vi "Variable list PSU analog.vi"() -> (6 "Variant":variant, 10 "Array":T1[](array[typedef]) {"Default Scaling"."Offset" format="%.5f"; "Default Scaling"."Gain" format="%.5f"})   [LabVIEW 2011]
uses:
  Measurments Handling/Fixed Analog Channel Definition.ctl
  Measurments Handling/Units/Quantity enum.ctl
  Measurments Handling/Update frequensies.ctl
  Measurments Handling/Channel catagory Enum.ctl
  Measurments Handling/Scaling.ctl
  Measurments Handling/Channel Classification Enum.ctl
  Measurments Handling/Common/Variable List Common Analog.ctl
  <vilib>/Utility/VariantDataType/GetNumericInfo.vi
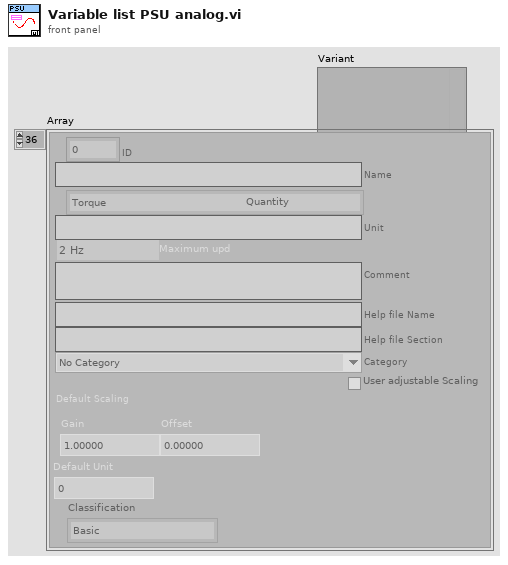
[diagram p1: front panel]
types:
  T1 = typedef "Fixed Analog Channel Definition.ctl" = cluster{"ID":u16, "Name":string, "Quantity":T2, "Unit":string, "Maximum upd":T3, "Comment":string, "Help file Name":string, "Help file Section ":string, "Category":T4, "User adjustable Scaling":bool, "Default Scaling":T5, "Default Unit":i32, "Classification":T6}
  T2 = typedef "Quantity enum.ctl" = enum16{"NA", "Acceleration", "Angle", "Current", "Force", "Distance", "Pressure", "Resistance", "Rotational Speed", "Speed", "Temperature", "Tension", "Torque", "Voltage", "Weight"}
  T3 = typedef "Update frequensies.ctl" = enum16{"2 Hz", "1 Hz", "0.1 Hz"}
  T4 = typedef "Channel catagory Enum.ctl" = enum16{"No Category", "Power", "Temperature", "Pressure"}
  T5 = typedef "Scaling.ctl" = cluster{"Gain":dbl, "Offset":dbl}
  T6 = typedef "Channel Classification Enum.ctl" = enum16{"Basic", "Advanced", "Expert", "Unused"}
  T7 = typedef "Variable List Common Analog.ctl" = enum16{"HVPSU Head Voltage", "HVPSU TS Voltage", "HVPSU Current", "PCP Cable Resistance", "Winch Depth", "Winch Line Speed", "Winch Wire Tension"}
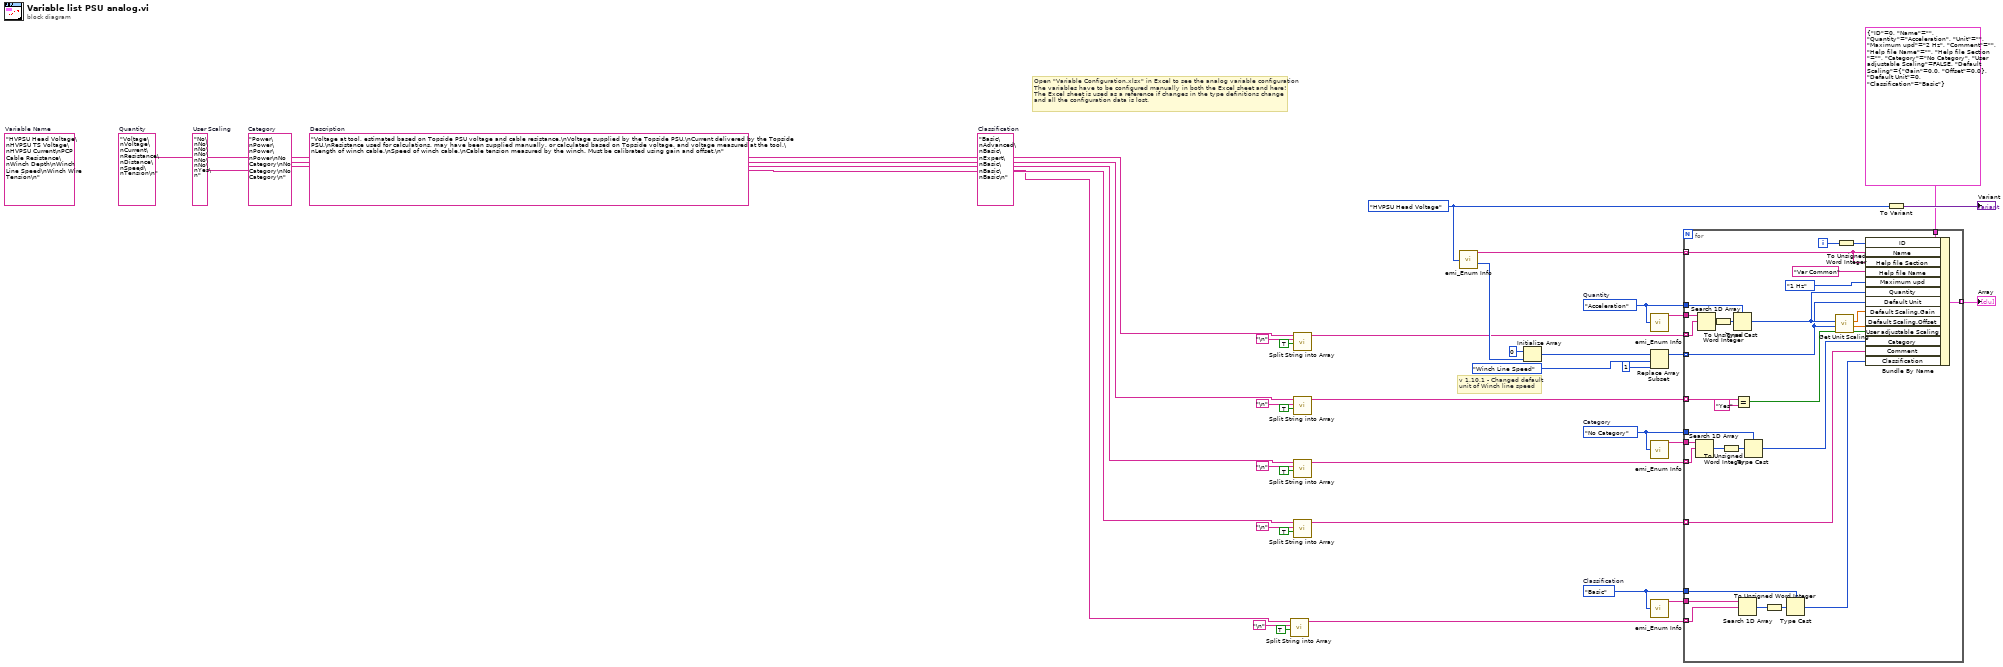
[diagram p0: block diagram]
diagram:
  w6 = Channel_Classification_Enum."Basic"  # Classification
  w7 = "Basic\nAdvanced\nBasic\nExpert\nBasic\nBasic\nBasic\n"  # Classification
  w3 = Variable_List_Common_Analog."HVPSU Head Voltage" ("Action")
  w12 = "Power\nPower\nPower\nPower\nNo Category\nNo Category\nNo Category\n"  # Category
  w15 = Channel_catagory_Enum."No Category"  # Category
  w18 = "No\nNo\nNo\nNo\nNo\nNo\nYes\n"  # User Scaling
  w23 = Quantity_enum."Acceleration"  # Quantity
  w10 = "Voltage\nVoltage\nCurrent\nResistance\nDistance\nSpeed\nTension\n"  # Quantity
  w22 = "Voltage at tool, estimated based on Topside PSU voltage and cable resistance.\nVoltage supplied by the Topside PSU.\nCurrent delivered by the Topside PSU.\nResistance used for calculations, may have been supplied manually, or calculated based on Topside voltage, and voltage measured at the tool.\nLength of winch cable.\nSpeed of winch cable.\nCable tension measured by the winch. Must be calibrated using gain and offset.\n"  # Description
  (unwired) "HVPSU Head Voltage\nHVPSU TS Voltage\nHVPSU Current\nPCP Cable Resistance\nWinch Depth\nWinch Line Speed\nWinch Wire Tension\n"  # Variable Name
  # "v 1.10.1 - Changed default \nunit of Winch line speed"
  # "Open \"Variable Configuration.xlsx\" in Excel to see the analog variable configuration\nThe variables have to be configured manually in both the Excel sheet and here!\nThe Excel sheet is used as a reference if changes in the type definitions change\nand all the configuration data is lost."
  n1 = call "Split String into Array.vi"("Remove Last Row"=TRUE, "Separator"="\n", "Input string"=w7) -> ("Array of cells"=w4:string[])  [unwired: 8 in]
  n2 = call "Split String into Array.vi"("Remove Last Row"=TRUE, "Separator"="\n", "Input string"=w10) -> ("Array of cells"=w25:string[])  [unwired: 8 in]
  n3 = call "Split String into Array.vi"("Remove Last Row"=TRUE, "Separator"="\n", "Input string"=w18) -> ("Array of cells"=w17:string[])  [unwired: 8 in]
  n4 = call "Split String into Array.vi"("Remove Last Row"=TRUE, "Separator"="\n", "Input string"=w12) -> ("Array of cells"=w11:string[])  [unwired: 8 in]
  n5 = call "Split String into Array.vi"("Remove Last Row"=TRUE, "Separator"="\n", "Input string"=w22) -> ("Array of cells"=w21:string[])  [unwired: 8 in]
  n6 = call "emi_Enum Info.vi"("Enum"=w3) -> ("Text Elements"=w2:string[], "Numb Elements"=w34:i32)  [unwired: 11 in, 2 out]
  n7 = Initialize Array(0, w34) -> (w32:i32[])
  n8 = call "emi_Enum Info.vi"("Enum"=w23) -> ("Text Elements"=w24:string[])  [unwired: 11 in, 3 out]
  n9 = Replace Array Subset(array=w32, new element=1 ("new element/subarray"), index=Variable_List_Common_Analog."Winch Line Speed" ("Action")) -> (w30:i32[])
  n10 = call "emi_Enum Info.vi"("Enum"=w15) -> ("Text Elements"=w16:string[])  [unwired: 11 in, 3 out]
  n11 = call "emi_Enum Info.vi"("Enum"=w6) -> ("Text Elements"=w5:string[])  [unwired: 11 in, 3 out]
  n12 = for {
    tunnel: [w69] -> w35 mode=indexing
    tunnel: T1 {"ID"=0, "Name"="", "Quantity"=enum."Acceleration", "Unit"="", "Maximum upd"=enum."2 Hz", "Comment"="", "Help file Name"="", "Help file Section "="", "Category"=enum."No Category", "User adjustable Scaling"=FALSE, "Default Scaling"={"Gain"=0.0, "Offset"=0.0}, "Default Unit"=0, "Classification"=enum."Basic"} ("Variable Defenition") -> [w68]
    tunnel: w21 -> [w51] mode=indexing
    tunnel: w30 -> [w58] mode=indexing
    tunnel: w25 -> [w65] mode=indexing
    tunnel: w24 -> [w66]
    tunnel: w23 -> [w63]
    tunnel: w17 -> [w57] mode=indexing
    tunnel: w11 -> [w53] mode=indexing
    tunnel: w16 -> [w52]
    tunnel: w15 -> [w54]
    tunnel: w4 -> [w43] mode=indexing
    tunnel: w5 -> [w44]
    tunnel: w6 -> [w42]
    tunnel: w2 -> [w38] mode=indexing
    i -> [w39]
    n13 = Search 1D Array(1D array=w52, element=w53) -> (index of element=w49:i32)  [unwired: 1 in]
    n14 = Search 1D Array(1D array=w66, element=w65) -> (index of element=w64:i32)  [unwired: 1 in]
    n15 = To Unsigned Word Integer(number=w64) -> (unsigned 16bit integer=w47:u16)
    n16 = To Unsigned Word Integer(number=w49) -> (unsigned 16bit integer=w48:u16)
    n17 = Type Cast(type=w63, x=w47) -> (*(type *) &x=w61:T2)
    n18 = Equal?(x=w57, y="Yes") -> (x = y?=w55:bool)
    n19 = Search 1D Array(1D array=w44, element=w43) -> (index of element=w45:i32)  [unwired: 1 in]
    n20 = Type Cast(type=w54, x=w48) -> (*(type *) &x=w50:T4)
    n21 = To Unsigned Word Integer(number=w45) -> (unsigned 16bit integer=w46:u16)
    n22 = Type Cast(type=w42, x=w46) -> (*(type *) &x=w41:T6)
    n23 = call "Get Unit Scaling.vi"("Unit Index"=w58, "Quantity"=w61) -> ("Offset"=w59:dbl, "Gain"=w60:dbl)  [unwired: 7 in, 1 out]
    n24 = To Unsigned Word Integer(number=w39) -> (unsigned 16bit integer=w40:u16)
    n25 = Bundle By Name(cluster=w68, "ID"=w40, "Name"=w38, "Help file Section"=w38, "Help file Name"="Var Common", "Maximum upd"=Update_frequensies."1 Hz", "Quantity"=w61, "Default Unit"=w58, "Default Scaling.Gain"=w60, "Default Scaling.Offset"=w59, "User adjustable Scaling"=w55, "Category"=w50, "Comment"=w51, "Classification"=w41) -> (w69:T1)
  }
  "Array" <- w35
  n26 = To Variant(anything=w3) -> (Variant=→"Variant":variant)
